vi "LET Output v3.vi"() -> ()   [LabVIEW 2010]
doc: "Cont(inuous) Acq(uire) & Chart (hw timed) demonstrates the hardware timed, non-buffered technique of data acquisition. The scan clock on the board controls acquisition timing. Acquired scans are read directly from the device's FIFO using AI Single Scan. \n\nThe acquisition is configured with no buffer, and the on-board scan clock started at the selected scan rate. In the first loop iteration, the newest (most recent) scan is read from the FIFO. In each subsequent loop iteration AI Single Scan is called to read the oldest scan from the FIFO. Then if a scan is missed because the acquisition does not keep up, an error message will be displayed, and the acquisition stopped. Each scan is plotted on the chart after it is read. \n\nA common reason to use non-buffered acquisition is that some kind of processing needs to be done for each data point. You will probably want to add more functions to the diagram to customize this VI for your application. The acquisition rate you can achieve depends on how much processing and display the VI must do. This VI calls a subVI named My Single-Scan Processing. Add whatever processing you need to this subVI, or replace it with one of your own. The data processing subVI also demonstrates how to use error clusters in your own subVIs, so they can be included in the error data flow chain.\n\nBefore running this VI, set the values of the controls on the front panel. Select Show Help Window from the Help menu to see a description of each control. If the values you select for all the controls are values you will usually use, select Make Current Values Default from the Operate menu and save the VI. Or, you may save individual control's default values by popping up on the control, selecting Data Operations, then selecting Make Current Value Default, and saving the VI."
uses:
  <instrlib>/agilent_b2900_series/Agilent B2900 Series/Public/Configure/Measurement/Configure Measurement (Current).vi
  <instrlib>/agilent_b2900_series/Agilent B2900 Series/Public/Configure/Measurement/Configure Measurement (Voltage).vi
  <vilib>/Analysis/Matrix/Numeric/Conversions/Matrix To Array - RM.vi
  <vilib>/Utility/file.llb/Write To Spreadsheet File (DBL).vi
  <instrlib>/agilent_b2900_series/Agilent B2900 Series/Agilent B2900 Series.lvlib
  <vilib>/Analysis/Matrix/NI_Matrix.lvlib
panel:
  out "Vds list":dbl[](array[numeric])
  out "Vgs list":dbl[](array[numeric])
  out "Real 2D Array":dbl[][](array[numeric])
  out "data matrix":dbl[][](array[numeric])
  out "Igs array 2":dbl[][](array[numeric])
  out "Vgs array 2":dbl[][](array[numeric])
  out "Vds array 2":dbl[][](array[numeric])
  out "Corrected PD current array 2":dbl[][](array[numeric])
  out "Ids array 2":dbl[][](array[numeric])
  out "corrected PD current array":dbl[](array[numeric])
  out "Vds array":dbl[](array[numeric])
  out "Ids array":dbl[](array[numeric])
  out "Vgs array":dbl[](array[numeric])
  out "Igs array":dbl[](array[numeric])
  in  "Tab Control":T1(tab)
  in  "keithley address":string="GPIB0::20::INSTR"
  in  "agilent address":refnum<visa-resource-name>="GPIB0::23::INSTR"
  in  "Initial Vds (V)\n(100 scans/sec)":sgl caption="Initial Vds (V)" format="%.2f"
  in  "Vds step (V)":sgl=1.0 format="%.2f"
  in  "Vds delay time":sgl=10.0 caption="Vds delay time (ms)" format="%.2f"
  in  "Vds delay after first value (ms)":sgl=10.0 format="%.2f"
  in  "Final Vds(V)":sgl=60.0 format="%.2f"
  in  "light emission ON/OFF":bool=TRUE
  in  "Vgs step (V)":sgl=20.0 format="%.2f"
  in  "Final Vgs (V)":sgl=60.0 format="%.2f"
  in  "Initial Vgs (V)":sgl format="%.2f"
  in  "Vgs hold time (ms)":i32=10
  in  "Compliance Voltage (channel 2)":dbl=60.0
  in  "Compliance Current (channel 1)":dbl=0.001
  in  "Compliance Voltage (channel 1)":dbl=60.0
  in  "Compliance Current (channel 2)":dbl=0.0001
  in  "keithley compliance limit":dbl(ring)=0.025 items=["25uA"=2.5e-05, "250uA"=0.00025, "2.5mA"=0.0025, "25mA"=0.025]
  in  "Loop":bool=TRUE
  in  "keithley current resolution":dbl=0.0001 format="%^.2e"
  in  "Current Auto Range Mode (0: Normal)":i32(ring) items=["Normal", "Resolution", "Speed"]
  in  "Voltage Auto Range Mode (0: Normal)":i32(ring) items=["Normal", "Resolution", "Speed"]
  in  "aperture time":dbl(ring)=-2.0 format="%.2f" items=["KE6485_VAL_RATE_FAST"=-1.0, "KE6485_VAL_RATE_MEDIUM"=-2.0, "KE6485_VAL_RATE_SLOW"=-3.0]
  in  "Auto Current NPLC (F: Disable)":bool
  in  "Current NPLC (0.1)":dbl=0.1
  in  "Auto Voltage NPLC(F: Disable)":bool
  in  "Voltage NPLC (0.1 PLC)":dbl=0.1
  out "Current Scan":cluster{dbl[], dbl[]}(graph)
  out "Applied Vds":sgl caption="current VDS (V)" format="%.2f"
  out "Applied Vgs":sgl caption="current VDS (V)" format="%.2f"
  out "Measured Ids":dbl format="%.2e"
  out "Measured Vds":dbl
  out "corrected PD current":dbl format="%^.2e"
  out "dark PD current (A)":dbl format="%^.2e"
  out "PD current":dbl format="%^.2e"
  out "Measured Igs":dbl
  out "Measured Vgs":dbl
  out "channel 2 status":bool
  out "channel 1 status":bool
  out "Current Scan 2":cluster{dbl[], dbl[]}(graph) caption="Current Scan"
  out "half  points":sgl
  out "Vds points":sgl
  out "Vgs points":sgl
  out "?":cluster{dbl[], dbl[]}[](graph)
  out "?":cluster{dbl[], dbl[]}[](graph)
  in  "error in keithley":errorcluster
  out "keithley address out":refnum<k15>
  out "error out keithley":errorcluster
  out "error out agilent":errorcluster
  out "Agilent address out":refnum<visa-resource-name>
  # "FET output v3"
  # "Drain-Source Setting"
  # "Gate Setting"
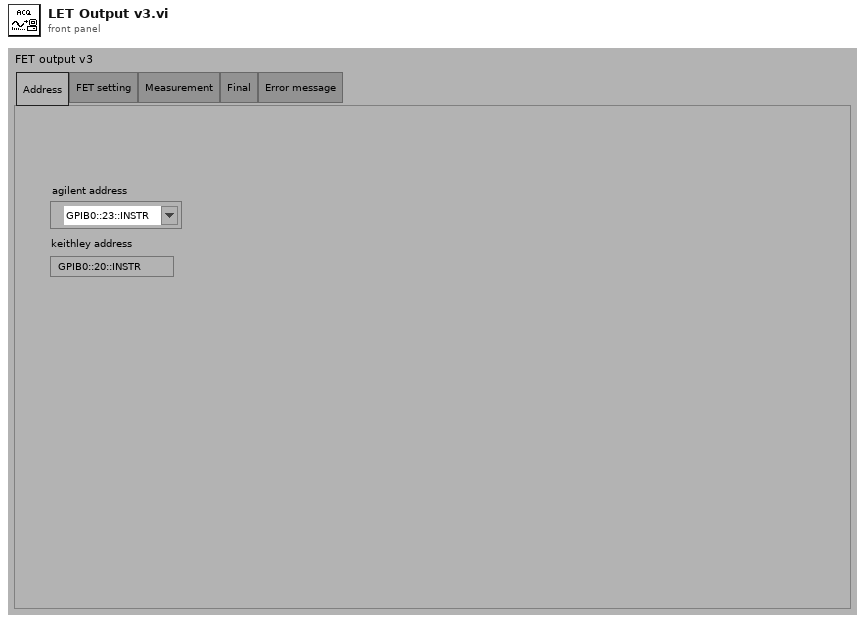
[diagram p1: front panel]
types:
  T1 = enum32{"Address", "FET setting", "Measurement", "Final", "Error message"}
  T2 = typedef "NI_Matrix.lvlib/RealMatrix.ctl" = dbl[][]
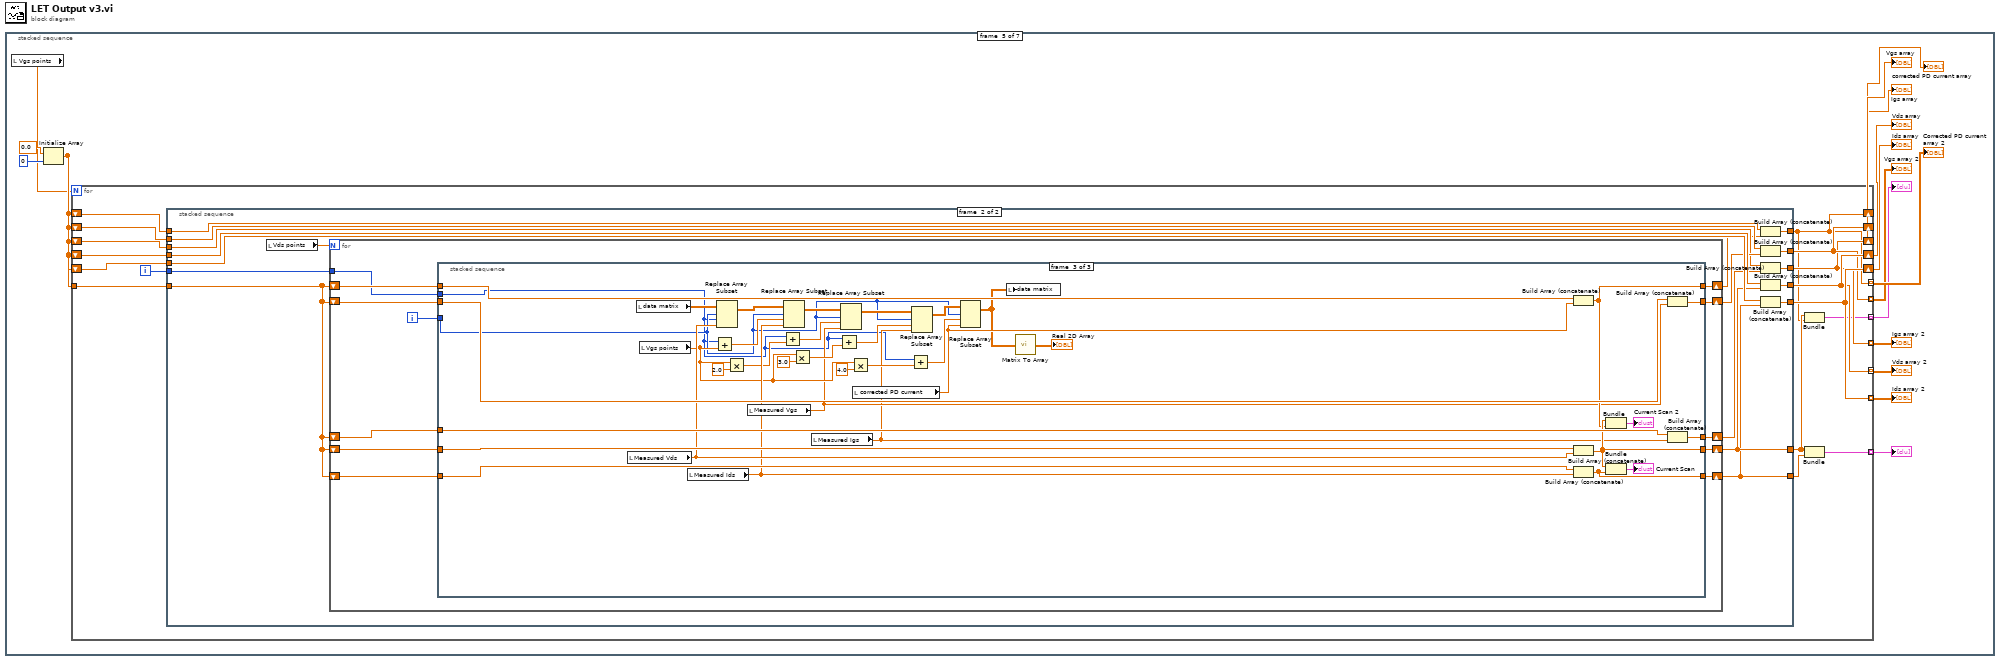
[diagram p0: block diagram]
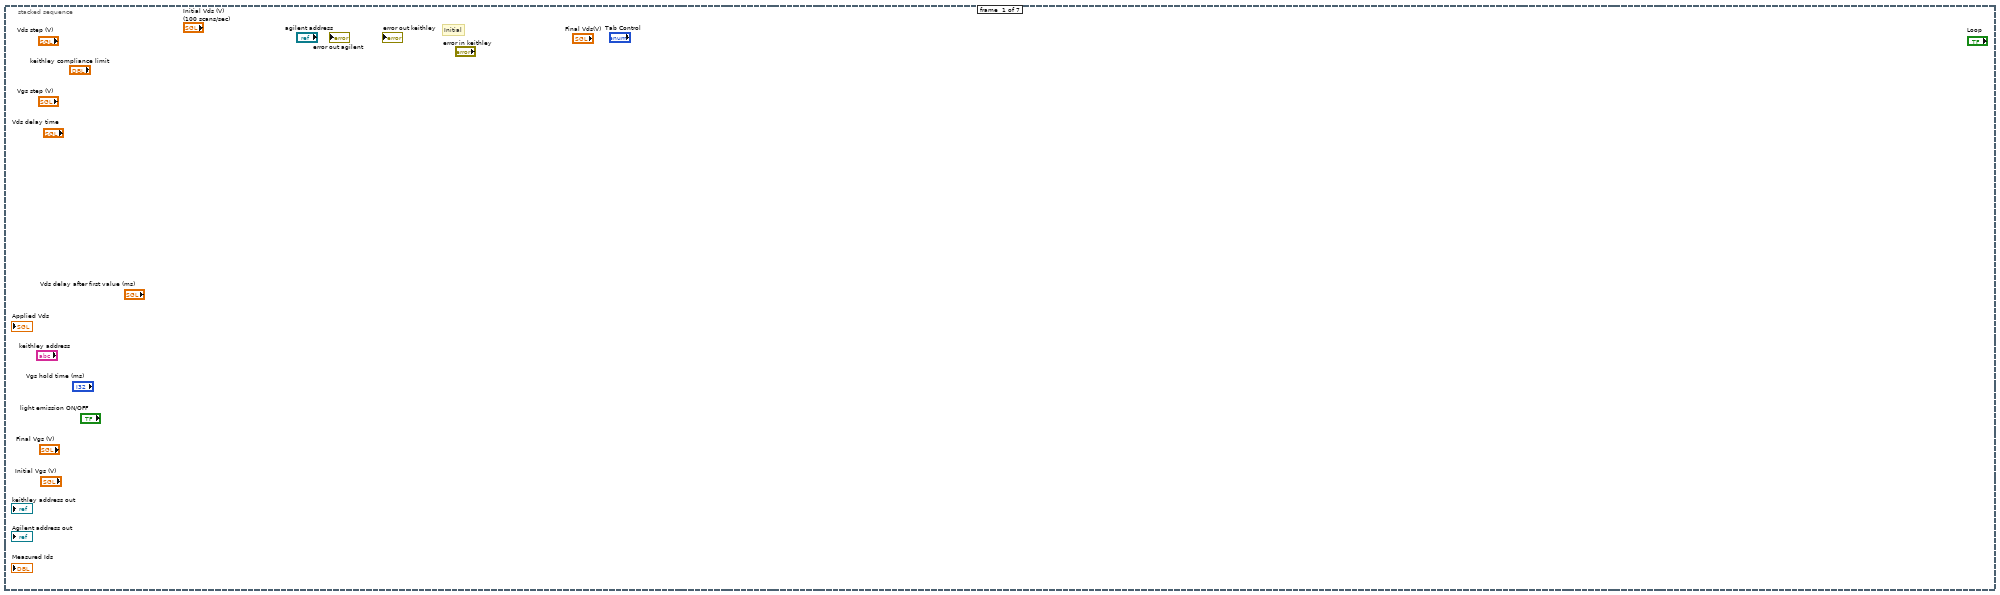
[diagram p2: hidden frame]
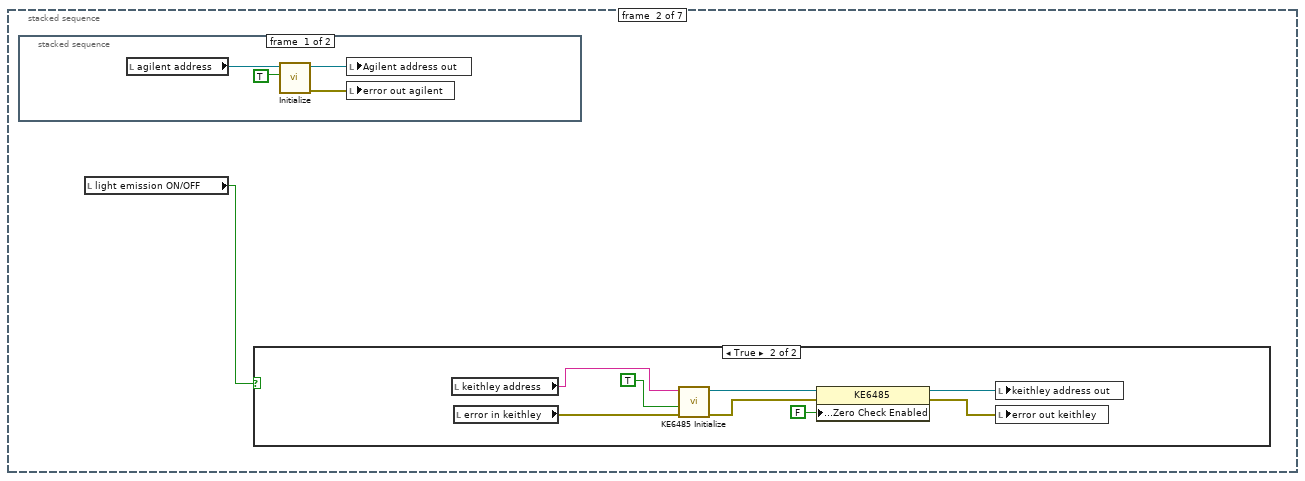
[diagram p3: hidden frame]
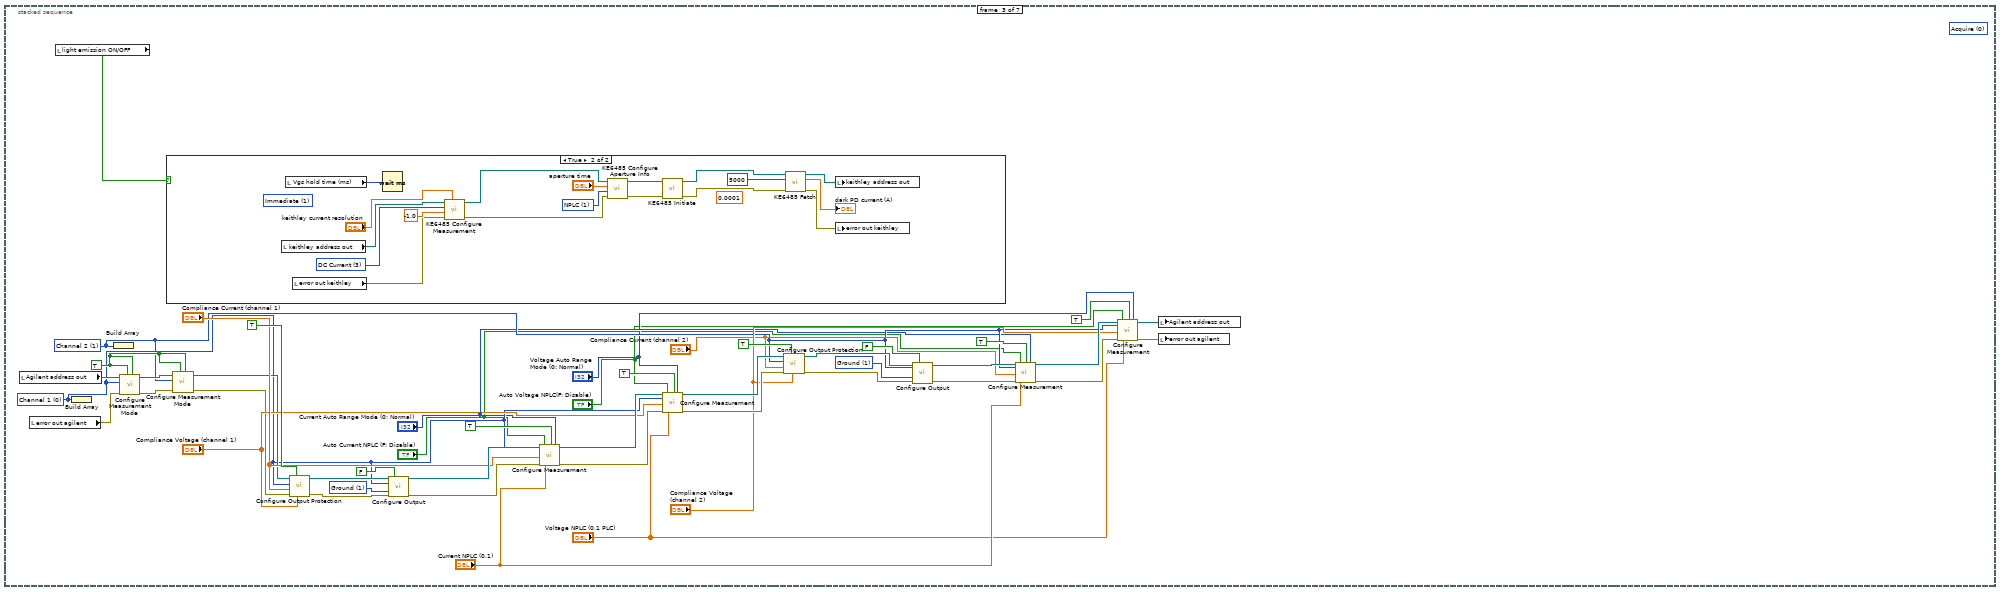
[diagram p6: hidden frame]
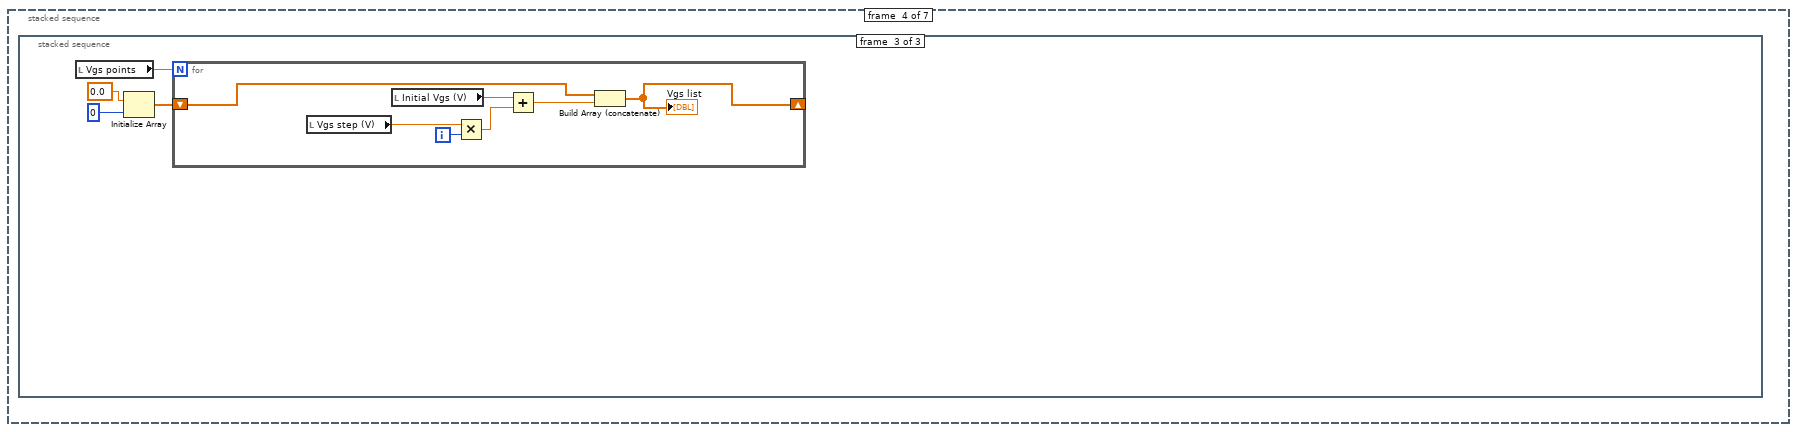
[diagram p8: hidden frame]
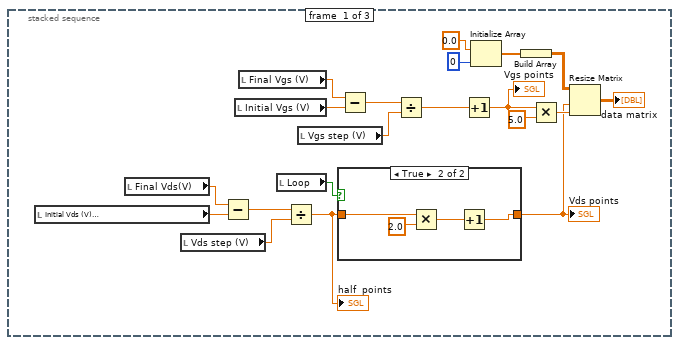
[diagram p9: hidden frame]
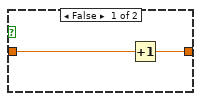
[diagram p10: hidden frame]
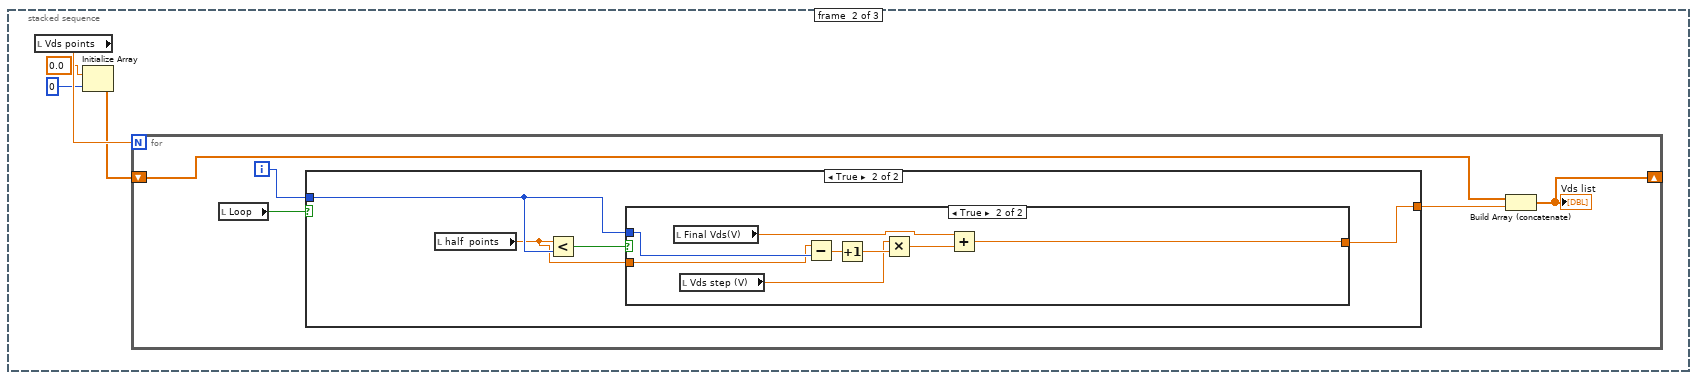
[diagram p11: hidden frame]
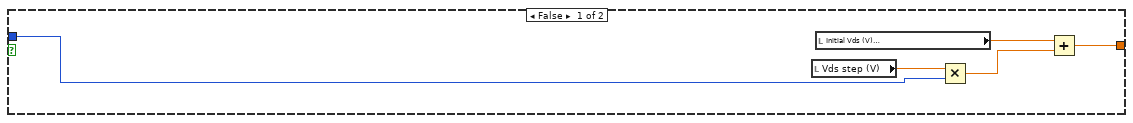
[diagram p12: hidden frame]
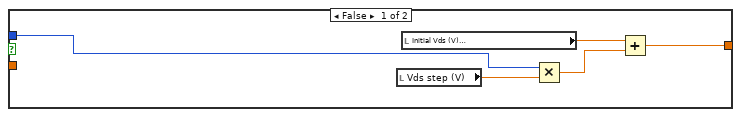
[diagram p13: hidden frame]
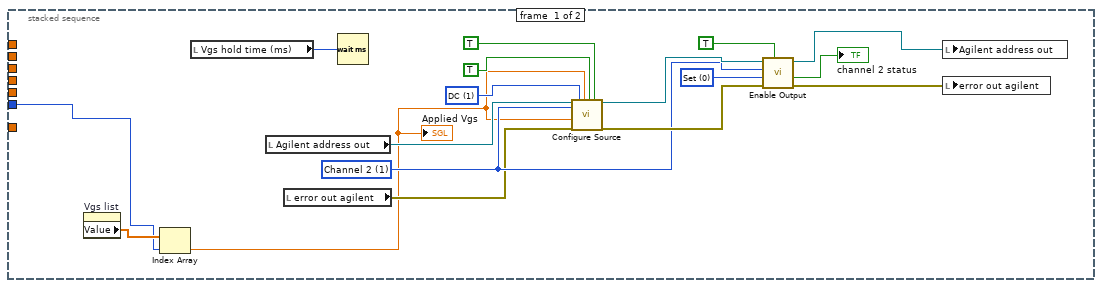
[diagram p14: hidden frame]
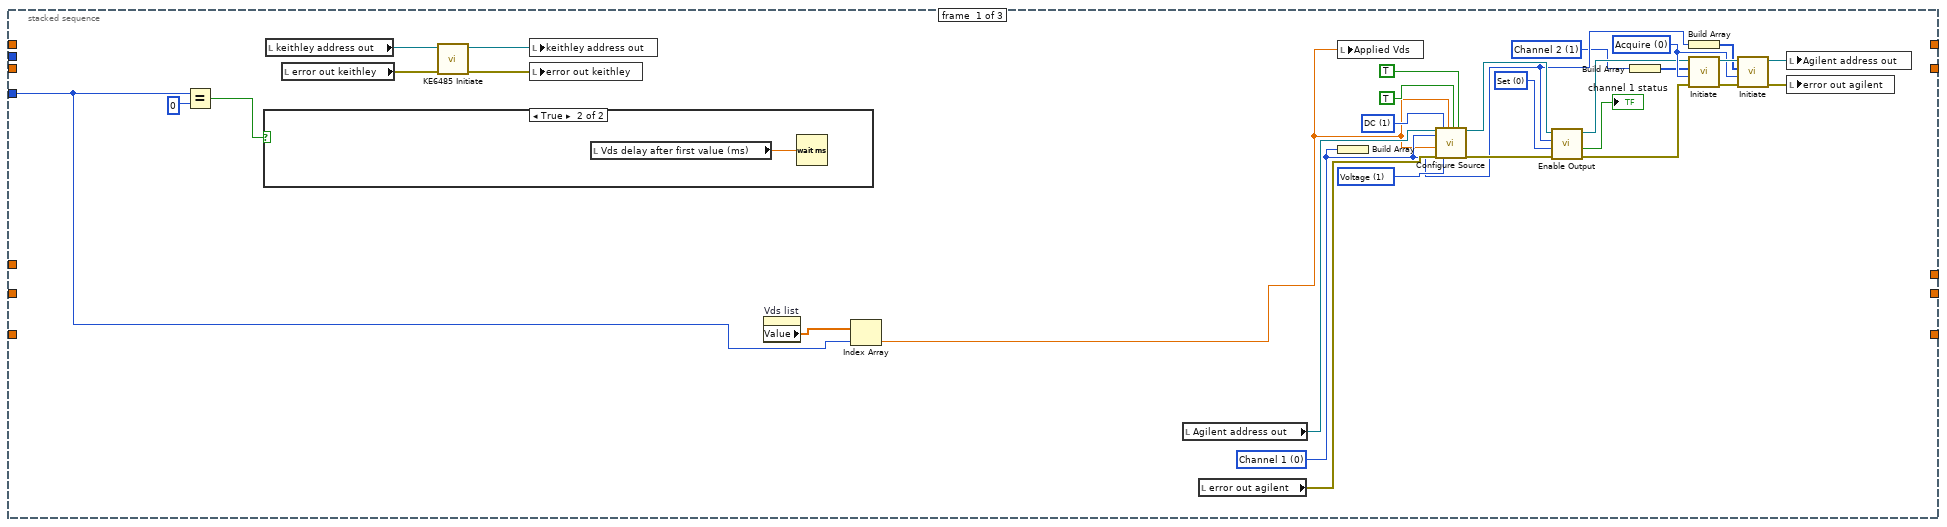
[diagram p15: hidden frame]
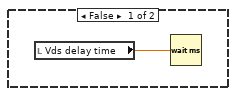
[diagram p16: hidden frame]
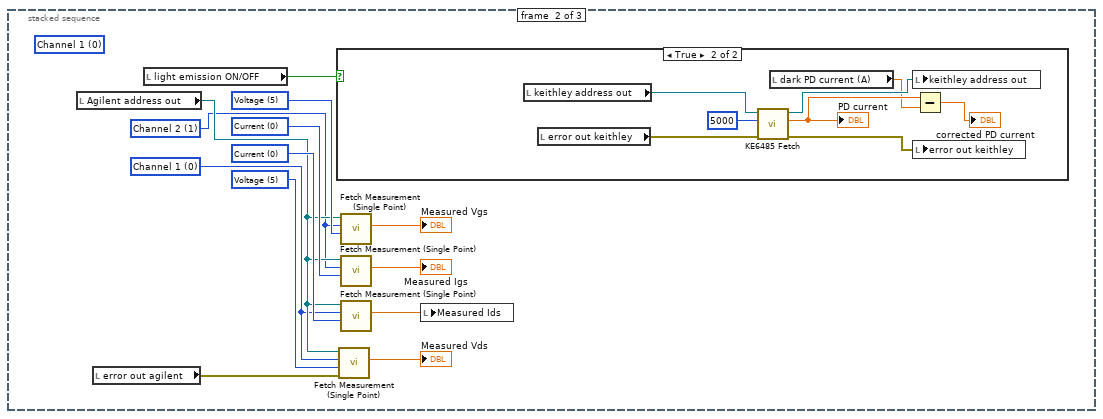
[diagram p17: hidden frame]
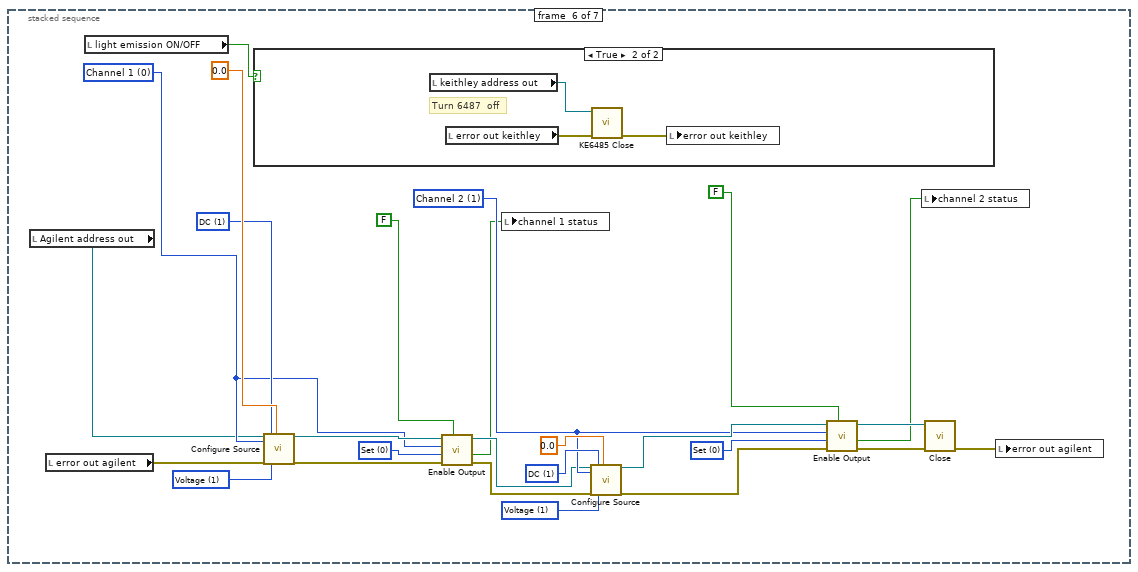
[diagram p19: hidden frame]
diagram:
  n1 = stacked-sequence {
    frame #0 {
      # "Initial"
    }
    frame #1 {
      n2 = stacked-sequence {
        frame #0 {
          n3 = local read "agilent address"() -> (w2:refnum<visa-resource-name>)
          n4 = call <instrlib>:"Initialize.vi"("ID Query (True)"=TRUE, "VISA resource name"=w2) -> ("error out"=w3:errorcluster, "VISA resource name out"=w4:refnum<visa-resource-name>)  [unwired: 8 in]
          n5 = local write "Agilent address out"(w4) -> ()
          n6 = local write "error out agilent"(w3) -> ()
        }
        frame #1 {
        }
      }
      n7 = local read "light emission ON/OFF"() -> (w1:bool)
      n8 = case shown="True" w1 {
        frame False {
        }
        frame True {
          n9 = local read "keithley address"() -> (w12:string)
          n10 = local read "error in keithley"() -> (w13:errorcluster)
          n11 = call <instrlib>:"KE6485 Initialize.vi"("error in (no error)"=w13, "reset device"=TRUE, "resource name"=w12) -> ("error out"=w10:errorcluster, "instrument handle out"=w9:refnum<k15>)  [unwired: 1 in, 6 out]
          n12 = property class="KE6485"(reference=w9, error in=w10, "System Settings:Zero Check Enabled"=FALSE) -> (reference out=w8:refnum<k15>, error out=w7:errorcluster)
          n13 = local write "keithley address out"(w8) -> ()
          n14 = local write "error out keithley"(w7) -> ()
        }
      }
    }
    frame #2 {
      (unwired) 0 items=["Acquire", "Transient", "Both"] ("Device Action (2: Both)")
      w30 = TRUE ("Enable Voltage Measurement (T: Enable)")
      w42 = 1 items=["Float", "Ground"] ("Low Terminal State (1: Ground)")
      w22 = 1 items=["Channel 1", "Channel 2"] ("Channel (0: Channel 1)")
      w52 = 1 items=["Float", "Ground"] ("Low Terminal State (1: Ground)")
      w23 = 0 items=["Channel 1", "Channel 2"] ("Channel (0: Channel 1)")
      n15 = local read "Agilent address out"() -> (w25:refnum<visa-resource-name>)
      n16 = local read "error out agilent"() -> (w27:errorcluster)
      n17 = local read "light emission ON/OFF"() -> (w59:bool)
      n18 = Build Array(w23) -> ()  [unwired: 1 out]
      n19 = Build Array(w22) -> ()  [unwired: 1 out]
      n20 = call <instrlib>:"Configure Measurement Mode.vi"("Enable Current Measurement (T: Enable)"=w30, "Enable Voltage Measurement (T: Enable)"=w30, "error in (no error)"=w27, "Channel (0: Channel 1)"=w23, "VISA resource name"=w25) -> ("error out"=w28:errorcluster, "VISA resource name out"=w29:refnum<visa-resource-name>)  [unwired: 5 in]
      n21 = case shown="True" w59 {
        frame False {
        }
        frame True {
          w65 = 1 items=["NPLC"=1] ("aperture time unit")
          (unwired) 0.0001 ("resolution (absolute)")
          (unwired) 1 items=["Immediate"=1, "Interval"=10, "Trigger Link 1"=1001, "Trigger Link 2"=1002, "Trigger Link 3"=1003, "Trigger Link 4"=1004, "Trigger Link 5"=1005, "Trigger Link 6"=1006] ("sample trigger")
          w75 = 3 items=["DC Volts"=1, "DC Current"=3, "2 Wire Resistance"=5, "Charge"=1004] ("measurement function")
          n22 = local read "keithley address out"() -> (w70:refnum<k15>)
          n23 = local read "Vgs hold time (ms)"() -> (w77:i32)
          n24 = local read "error out keithley"() -> (w69:errorcluster)
          n25 = Wait (ms)(milliseconds to wait=w77) -> ()  [unwired: 1 out]
          n26 = call <instrlib>:"KE6485 Configure Measurement.vi"("resolution (absolute)"="keithley current resolution", "error in (no error)"=w69, "range"=-1.0, "measurement function"=w75, "instrument handle"=w70) -> ("error out"=w64:errorcluster, "instrument handle out"=w63:refnum<k15>)  [unwired: 5 in]
          n27 = call <instrlib>:"KE6485 Configure Aperture Info.vi"("error in (no error)"=w64, "aperture time unit"=w65, "aperture time"="aperture time", "instrument handle"=w63) -> ("error out"=w61:errorcluster, "instrument handle out"=w62:refnum<k15>)  [unwired: 6 in]
          n28 = call <instrlib>:"KE6485 Initiate.vi"("error in (no error)"=w61, "instrument handle"=w62) -> ("error out"=w67:errorcluster, "instrument handle out"=w68:refnum<k15>)  [unwired: 8 in]
          n29 = call <instrlib>:"KE6485 Fetch.vi"("error in (no error)"=w67, "maximum time (ms)"=5000, "instrument handle"=w68) -> ("error out"=w72:errorcluster, "reading"=→"dark PD current (A)":dbl, "instrument handle out"=w71:refnum<k15>)  [unwired: 6 in]
          n30 = local write "keithley address out"(w71) -> ()
          n31 = local write "error out keithley"(w72) -> ()
        }
      }
      n32 = call <instrlib>:"Configure Measurement Mode.vi"("Enable Current Measurement (T: Enable)"=w30, "Enable Voltage Measurement (T: Enable)"=w30, "error in (no error)"=w28, "Channel (0: Channel 1)"=w22, "VISA resource name"=w29) -> ("error out"=w26:errorcluster, "VISA resource name out"=w24:refnum<visa-resource-name>)  [unwired: 5 in]
      n33 = call <instrlib>:"Configure Output Protection.vi"("Compliance Voltage (2 V)"="Compliance Voltage (channel 1)", "Enable Output Protection (T: Enable)"=TRUE, "error in (no error)"=w26, "Compliance Current (0.0001 A)"="Compliance Current (channel 1)", "Channel (0: Channel 1)"=w23, "VISA resource name"=w24) -> ("error out"=w54:errorcluster, "VISA resource name out"=w53:refnum<visa-resource-name>)  [unwired: 4 in]
      n34 = call <instrlib>:"Configure Output.vi"("VISA resource name"=w53, "Auto Output-Off (F: Disable)"=FALSE, "Channel (0: Channel 1)"=w23, "Low Terminal State (1: Ground)"=w52, "error in (no error)"=w54) -> ("VISA resource name out"=w50:refnum<visa-resource-name>, "error out"=w51:errorcluster)  [unwired: 9 in]
      n35 = call-poly <instrlib>:"Configure Measurement.vi"("VISA resource name"=w50, "Channel (0: Channel 1)"=w23, "Current Range (0.0001 A)"="Compliance Current (channel 1)", "error in (no error)"=w51, "Auto Current NPLC (F: Disable)"="Auto Current NPLC (F: Disable)", "Current NPLC (0.1)"="Current NPLC (0.1)", "Current Auto Range (T: Enable)"=TRUE, "Current Auto Range Mode (0: Normal)"="Current Auto Range Mode (0: Normal)") -> ("VISA resource name out"=w58:refnum<visa-resource-name>, "error out"=w57:errorcluster)  [unwired: 10 in]
      n36 = call-poly <instrlib>:"Configure Measurement.vi"("VISA resource name"=w58, "Channel (0: Channel 1)"=w23, "Voltage Range (2 V)"="Compliance Voltage (channel 1)", "error in (no error)"=w57, "Auto Voltage NPLC(F: Disable)"="Auto Voltage NPLC(F: Disable)", "Voltage NPLC (0.1 PLC)"="Voltage NPLC (0.1 PLC)", "Voltage Auto Range (T: Enable)"=TRUE, "Voltage Auto Range Mode (0: Normal)"="Voltage Auto Range Mode (0: Normal)") -> ("VISA resource name out"=w38:refnum<visa-resource-name>, "error out"=w37:errorcluster)  [unwired: 10 in]
      n37 = call <instrlib>:"Configure Output Protection.vi"("Compliance Voltage (2 V)"="Compliance Voltage (channel 2)", "Enable Output Protection (T: Enable)"=TRUE, "error in (no error)"=w37, "Compliance Current (0.0001 A)"="Compliance Current (channel 2)", "Channel (0: Channel 1)"=w22, "VISA resource name"=w38) -> ("error out"=w44:errorcluster, "VISA resource name out"=w43:refnum<visa-resource-name>)  [unwired: 4 in]
      n38 = call <instrlib>:"Configure Output.vi"("VISA resource name"=w43, "Auto Output-Off (F: Disable)"=FALSE, "Channel (0: Channel 1)"=w22, "Low Terminal State (1: Ground)"=w42, "error in (no error)"=w44) -> ("VISA resource name out"=w40:refnum<visa-resource-name>, "error out"=w41:errorcluster)  [unwired: 9 in]
      n39 = call-poly <instrlib>:"Configure Measurement.vi"("VISA resource name"=w40, "Channel (0: Channel 1)"=w22, "Current Range (0.0001 A)"="Compliance Current (channel 2)", "error in (no error)"=w41, "Auto Current NPLC (F: Disable)"="Auto Current NPLC (F: Disable)", "Current NPLC (0.1)"="Current NPLC (0.1)", "Current Auto Range (T: Enable)"=TRUE, "Current Auto Range Mode (0: Normal)"="Current Auto Range Mode (0: Normal)") -> ("VISA resource name out"=w48:refnum<visa-resource-name>, "error out"=w47:errorcluster)  [unwired: 10 in]
      n40 = call-poly <instrlib>:"Configure Measurement.vi"("VISA resource name"=w48, "Channel (0: Channel 1)"=w22, "Voltage Range (2 V)"="Compliance Voltage (channel 2)", "error in (no error)"=w47, "Auto Voltage NPLC(F: Disable)"="Auto Voltage NPLC(F: Disable)", "Voltage NPLC (0.1 PLC)"="Voltage NPLC (0.1 PLC)", "Voltage Auto Range (T: Enable)"=TRUE, "Voltage Auto Range Mode (0: Normal)"="Voltage Auto Range Mode (0: Normal)") -> ("VISA resource name out"=w21:refnum<visa-resource-name>, "error out"=w20:errorcluster)  [unwired: 10 in]
      n41 = local write "Agilent address out"(w21) -> ()
      n42 = local write "error out agilent"(w20) -> ()
    }
    frame #3 {
      n43 = stacked-sequence {
        frame #0 {
          n44 = local read "Initial Vds (V)\n(100 scans/sec)"() -> (w82:sgl)
          n45 = local read "Final Vds(V)"() -> (w81:sgl)
          n46 = local read "Vds step (V)"() -> (w83:sgl)
          n47 = Subtract(x=w81, y=w82) -> (x-y=w84:sgl)
          n48 = local read "Initial Vgs (V)"() -> (w95:sgl)
          n49 = local read "Final Vgs (V)"() -> (w94:sgl)
          n50 = local read "Loop"() -> (w80:bool)
          n51 = Divide(x=w84, y=w83) -> (x/y=w79:sgl)
          "half  points" <- w79
          n52 = local read "Vgs step (V)"() -> (w96:sgl)
          n53 = case shown="True" w80 {
            tunnel: w79 -> [w99 w103]
            tunnel: [w98 w101] -> w78
            frame False {
              n54 = Increment(x=w99) -> (x+1=w98:sgl)
            }
            frame True {
              n55 = Multiply(x=w103, y=sgl 2.0) -> (x*y=w100:sgl)
              n56 = Increment(x=w100) -> (x+1=w101:sgl)
            }
          }
          "Vds points" <- w78
          n57 = Subtract(x=w94, y=w95) -> (x-y=w92:sgl)
          n58 = Divide(x=w92, y=w96) -> (x/y=w93:sgl)
          n59 = Increment(x=w93) -> (x+1=w97:sgl)
          "Vgs points" <- w97
          n60 = Initialize Array(0.0 ("element"), 0 ("dimension size")) -> (w87:dbl[])
          n61 = Build Array(w87) -> (w88:T2)
          n62 = Multiply(x=w97, y=sgl 5.0) -> (x*y=w91:sgl)
          n63 = Resize Matrix(1:w91, 2:w78, 4:w88) -> (0:→"data matrix":T2)
        }
        frame #1 {
          n64 = local read "Vds points"() -> (w107:sgl)
          n65 = Initialize Array(0.0, 0) -> (w104:dbl[])
          n66 = for {
            N: w107 -> [_]
            shift-right: [w109] -> _
            shift-left: w104 -> [w110]
            i -> [w111]
            n67 = local read "Loop"() -> (w112:bool)
            n68 = case shown="True" w112 {
              tunnel: w111 -> [w115 w120]
              tunnel: [w113 w121] -> w108
              frame False {
                n69 = local read "Vds step (V)"() -> (w116:sgl)
                n70 = local read "Initial Vds (V)\n(100 scans/sec)"() -> (w114:sgl)
                n71 = Multiply(x=w116, y=w115) -> (x*y=w117:sgl)
                n72 = Add(x=w114, y=w117) -> (x+y=w113:sgl)
              }
              frame True {
                n73 = local read "half  points"() -> (w118:sgl)
                n74 = Less?(x=w118, y=w120) -> (x < y?=w119:bool)
                n75 = case shown="True" w119 {
                  tunnel: w120 -> [w124 w130]
                  tunnel: [w122 w127] -> w121
                  tunnel: w118 -> [_ w129]
                  frame False {
                    n76 = local read "Vds step (V)"() -> (w123:sgl)
                    n77 = local read "Initial Vds (V)\n(100 scans/sec)"() -> (w125:sgl)
                    n78 = Multiply(x=w124, y=w123) -> (x*y=w126:sgl)
                    n79 = Add(x=w125, y=w126) -> (x+y=w122:sgl)
                  }
                  frame True {
                    n80 = local read "Final Vds(V)"() -> (w131:sgl)
                    n81 = local read "Vds step (V)"() -> (w128:sgl)
                    n82 = Subtract(x=w129, y=w130) -> (x-y=w133:sgl)
                    n83 = Increment(x=w133) -> (x+1=w132:sgl)
                    n84 = Multiply(x=w128, y=w132) -> (x*y=w134:sgl)
                    n85 = Add(x=w131, y=w134) -> (x+y=w127:sgl)
                  }
                }
              }
            }
            n86 = Build Array (concatenate)(w110, w108) -> (w109:dbl[])
            "Vds list" <- w109
          }
        }
        frame #2 {
          n87 = local read "Vgs points"() -> (w138:sgl)
          n88 = Initialize Array(0.0, 0) -> (w135:dbl[])
          n89 = for {
            N: w138 -> [_]
            shift-right: [w144] -> _
            shift-left: w135 -> [w145]
            i -> [w140]
            n90 = local read "Vgs step (V)"() -> (w143:sgl)
            n91 = local read "Initial Vgs (V)"() -> (w142:sgl)
            n92 = Multiply(x=w143, y=w140) -> (x*y=w141:sgl)
            n93 = Add(x=w142, y=w141) -> (x+y=w139:sgl)
            n94 = Build Array (concatenate)(w145, w139) -> (w144:dbl[])
            "Vgs list" <- w144
          }
        }
      }
    }
    frame #4 {
      n95 = local read "Vgs points"() -> (w146:sgl)
      n96 = Initialize Array(0.0, 0) -> (w153:dbl[])
      n97 = for {
        N: w146 -> [_]
        shift-right: [w168] -> w158
        shift-left: w153 -> [w176]
        shift-right: [w169] -> w159
        shift-left: w153 -> [w175]
        shift-right: [w166] -> w157
        shift-left: w153 -> [w174]
        tunnel: [w173] -> w156 mode=indexing
        shift-right: [w165] -> w155
        shift-left: w153 -> [w172]
        shift-right: [w163] -> w154
        shift-left: w153 -> [w171]
        tunnel: w153 -> [w170]
        tunnel: [w169] -> w152 mode=indexing
        tunnel: [w163] -> w151 mode=indexing
        tunnel: [w168] -> w150 mode=indexing
        tunnel: [w166] -> w149 mode=indexing
        tunnel: [w165] -> w148 mode=indexing
        tunnel: [w162] -> w147 mode=indexing
        i -> [w177]
        n98 = stacked-sequence {
          tunnel: w177 -> [w179 w195]
          tunnel: w176 -> [_ w212]
          tunnel: w175 -> [_ w211]
          tunnel: [_ w206] -> w168
          tunnel: [_ w210] -> w169
          tunnel: w174 -> [_ w208]
          tunnel: [_ w207] -> w166
          tunnel: [_ w205] -> w164
          tunnel: [_ w204] -> w167
          tunnel: w172 -> [_ w203]
          tunnel: [_ w202] -> w165
          tunnel: [_ w200] -> w163
          tunnel: w171 -> [_ w198]
          tunnel: w170 -> [_ w196]
          frame #0 {
            w187 = 0 items=["Set", "Get"] ("Operation (0: Set)")
            w188 = 1 items=["Channel 1", "Channel 2"] ("Channel (0: Channel 1)")
            w191 = 1 items=["Pulse", "DC"] ("Source Shape (1: DC)")
            n99 = property on="Vgs list" class="Arr (strict)"() -> ("Value"=w180:dbl[])  [unwired: 2 in, 2 out]
            n100 = Index Array(array=w180, index=w179) -> (element=w178:dbl)
            "Applied Vgs" <- w178
            n101 = local read "Vgs hold time (ms)"() -> (w194:i32)
            n102 = local read "Agilent address out"() -> (w184:refnum<visa-resource-name>)
            n103 = local read "error out agilent"() -> (w183:errorcluster)
            n104 = Wait (ms)(milliseconds to wait=w194) -> ()  [unwired: 1 out]
            n105 = call <instrlib>:"Configure Source.vi"("VISA resource name"=w184, "Channel (0: Channel 1)"=w188, "Source Range (2)"=w178, "error in (no error)"=w183, "Source Shape (1: DC)"=w191, "Output Level (0)"=w178, "Source Auto Range (T: Enable)"=TRUE, "Enable Continuous Output (T: Enable)"=TRUE) -> ("VISA resource name out"=w193:refnum<visa-resource-name>, "error out"=w192:errorcluster)  [unwired: 10 in]
            n106 = call <instrlib>:"Enable Output.vi"("Enable Output (T: Enable)"=TRUE, "error in (no error)"=w192, "Operation (0: Set)"=w187, "Channel (0: Channel 1)"=w188, "VISA resource name"=w193) -> ("error out"=w182:errorcluster, "Output Enabled?"=→"channel 2 status":bool, "VISA resource name out"=w181:refnum<visa-resource-name>)  [unwired: 4 in]
            n107 = local write "Agilent address out"(w181) -> ()
            n108 = local write "error out agilent"(w182) -> ()
          }
          frame #1 {
            n109 = local read "Vds points"() -> (w197:sgl)
            n110 = for {
              N: w197 -> [_]
              shift-right: [w215] -> w204
              shift-left: w196 -> [w214]
              shift-right: [w217] -> w205
              shift-left: w196 -> [w216]
              shift-right: [w221] -> w209
              shift-left: w196 -> [w220]
              shift-right: [w219] -> w201
              shift-left: w196 -> [w218]
              shift-right: [w222] -> w199
              shift-left: w196 -> [w223]
              tunnel: w195 -> [w213]
              i -> [w224]
              n111 = stacked-sequence {
                tunnel: w224 -> [w226 _ w279]
                tunnel: w223 -> [_ _ w314]
                tunnel: [_ _ w303] -> w222
                tunnel: [_ _ w313] -> w221
                tunnel: w220 -> [_ _ w312]
                tunnel: [_ _ w311] -> w219
                tunnel: w218 -> [_ _ w310]
                tunnel: [_ _ w304] -> w217
                tunnel: w216 -> [_ _ w308]
                tunnel: [_ _ w306] -> w215
                tunnel: w214 -> [_ _ w307]
                tunnel: w213 -> [_ _ w278]
                frame #0 {
                  w240 = 0 items=["Acquire", "Transient", "Both"] ("Device Action (2: Both)")
                  w232 = 1 items=["Channel 1", "Channel 2"] ("Channel (0: Channel 1)")
                  w243 = 1 items=["Current", "Voltage"] ("Source Mode (1: Voltage)")
                  w246 = 1 items=["Pulse", "DC"] ("Source Shape (1: DC)")
                  w233 = 0 items=["Channel 1", "Channel 2"] ("Channel (0: Channel 1)")
                  w250 = 0 items=["Set", "Get"] ("Operation (0: Set)")
                  n112 = Equal?(x=w226, y=0) -> (x = y?=w253:bool)
                  n113 = case shown="True" w253 {
                    frame False {
                      n114 = local read "Vds delay time"() -> (w255:sgl)
                      n115 = Wait (ms)(milliseconds to wait=w255) -> ()  [unwired: 1 out]
                    }
                    frame True {
                      n116 = local read "Vds delay after first value (ms)"() -> (w256:sgl)
                      n117 = Wait (ms)(milliseconds to wait=w256) -> ()  [unwired: 1 out]
                    }
                  }
                  n118 = local read "keithley address out"() -> (w229:refnum<k15>)
                  n119 = local read "error out keithley"() -> (w228:errorcluster)
                  n120 = call <instrlib>:"KE6485 Initiate.vi"("error in (no error)"=w228, "instrument handle"=w229) -> ("error out"=w231:errorcluster, "instrument handle out"=w230:refnum<k15>)  [unwired: 8 in]
                  n121 = local write "keithley address out"(w230) -> ()
                  n122 = local write "error out keithley"(w231) -> ()
                  n123 = property on="Vds list" class="Arr (strict)"() -> ("Value"=w227:dbl[])  [unwired: 2 in, 2 out]
                  n124 = Index Array(array=w227, index=w226) -> (element=w225:dbl)
                  n125 = local read "Agilent address out"() -> (w248:refnum<visa-resource-name>)
                  n126 = local read "error out agilent"() -> (w247:errorcluster)
                  n127 = local write "Applied Vds"(w225) -> ()
                  n128 = Build Array(w233) -> ()  [unwired: 1 out]
                  n129 = call <instrlib>:"Configure Source.vi"("VISA resource name"=w248, "Channel (0: Channel 1)"=w233, "Source Range (2)"=w225, "error in (no error)"=w247, "Source Shape (1: DC)"=w246, "Source Mode (1: Voltage)"=w243, "Output Level (0)"=w225, "Source Auto Range (T: Enable)"=TRUE, "Enable Continuous Output (T: Enable)"=TRUE) -> ("VISA resource name out"=w252:refnum<visa-resource-name>, "error out"=w251:errorcluster)  [unwired: 9 in]
                  n130 = call <instrlib>:"Enable Output.vi"("error in (no error)"=w251, "Operation (0: Set)"=w250, "Channel (0: Channel 1)"=w233, "VISA resource name"=w252) -> ("error out"=w236:errorcluster, "Output Enabled?"=→"channel 1 status":bool, "VISA resource name out"=w237:refnum<visa-resource-name>)  [unwired: 5 in]
                  n131 = Build Array(w232) -> (w239:i32[])
                  n132 = Build Array(w233) -> (w238:i32[])
                  n133 = call <instrlib>:"Initiate.vi"("error in (no error)"=w236, "Device Action (2: Both)"=w240, "Channel List ({Channel1})"=w239, "VISA resource name"=w237) -> ("error out"=w242:errorcluster, "VISA resource name out"=w241:refnum<visa-resource-name>)  [unwired: 6 in]
                  n134 = call <instrlib>:"Initiate.vi"("error in (no error)"=w242, "Device Action (2: Both)"=w240, "Channel List ({Channel1})"=w238, "VISA resource name"=w241) -> ("error out"=w235:errorcluster, "VISA resource name out"=w234:refnum<visa-resource-name>)  [unwired: 6 in]
                  n135 = local write "Agilent address out"(w234) -> ()
                  n136 = local write "error out agilent"(w235) -> ()
                }
                frame #1 {
                  w258 = 1 items=["Channel 1", "Channel 2"] ("Channel (0: Channel 1)")
                  w259 = 0 items=["Channel 1", "Channel 2"] ("Channel (0: Channel 1)")
                  w264 = 0 items=["Current", "Resistance", "Source Output Setting", "Status", "Time", "Voltage"] ("Data Mode (5: Voltage)")
                  w265 = 5 items=["Current", "Resistance", "Source Output Setting", "Status", "Time", "Voltage"] ("Data Mode (5: Voltage)")
                  w267 = 0 items=["Current", "Resistance", "Source Output Setting", "Status", "Time", "Voltage"] ("Data Mode (5: Voltage)")
                  (unwired) 0 items=["Channel 1", "Channel 2"] ("Channel (0: Channel 1)")
                  w269 = 5 items=["Current", "Resistance", "Source Output Setting", "Status", "Time", "Voltage"] ("Data Mode (5: Voltage)")
                  n137 = local read "Agilent address out"() -> (w260:refnum<visa-resource-name>)
                  n138 = local read "error out agilent"() -> (w261:errorcluster)
                  n139 = local read "light emission ON/OFF"() -> (w257:bool)
                  n140 = case shown="True" w257 {
                    frame False {
                    }
                    frame True {
                      n141 = local read "keithley address out"() -> (w271:refnum<k15>)
                      n142 = local read "error out keithley"() -> (w270:errorcluster)
                      n143 = call <instrlib>:"KE6485 Fetch.vi"("error in (no error)"=w270, "maximum time (ms)"=5000, "instrument handle"=w271) -> ("error out"=w276:errorcluster, "reading"=w273:dbl, "instrument handle out"=w275:refnum<k15>)  [unwired: 6 in]
                      "PD current" <- w273
                      n144 = local read "dark PD current (A)"() -> (w272:dbl)
                      n145 = local write "keithley address out"(w275) -> ()
                      n146 = local write "error out keithley"(w276) -> ()
                      n147 = Subtract(x=w273, y=w272) -> (x-y=→"corrected PD current":dbl)
                    }
                  }
                  n148 = call <instrlib>:"Fetch Measurement (Single Point).vi"("error in (no error)"=w261, "Data Mode (5: Voltage)"=w269, "Channel (0: Channel 1)"=w259, "VISA resource name"=w260) -> ("Measurement"=→"Measured Vds":dbl)  [unwired: 5 in, 2 out]
                  n149 = call <instrlib>:"Fetch Measurement (Single Point).vi"("Data Mode (5: Voltage)"=w265, "Channel (0: Channel 1)"=w258, "VISA resource name"=w260) -> ("Measurement"=→"Measured Vgs":dbl)  [unwired: 6 in, 2 out]
                  n150 = call <instrlib>:"Fetch Measurement (Single Point).vi"("Data Mode (5: Voltage)"=w264, "Channel (0: Channel 1)"=w258, "VISA resource name"=w260) -> ("Measurement"=→"Measured Igs":dbl)  [unwired: 6 in, 2 out]
                  n151 = call <instrlib>:"Fetch Measurement (Single Point).vi"("Data Mode (5: Voltage)"=w267, "Channel (0: Channel 1)"=w259, "VISA resource name"=w260) -> ("Measurement"=w266:dbl)  [unwired: 6 in, 2 out]
                  n152 = local write "Measured Ids"(w266) -> ()
                }
                frame #2 {
                  n153 = local read "Measured Vds"() -> (w301:dbl)
                  n154 = local read "data matrix"() -> (w302:dbl[][])
                  n155 = local read "Vgs points"() -> (w285:sgl)
                  n156 = local read "Measured Ids"() -> (w298:dbl)
                  n157 = Add(x=w278, y=w285) -> (x+y=w299:sgl)
                  n158 = Replace Array Subset(array=w302, new element=w301, index (row)=w279, index (col)=w278) -> (w300:T2)
                  n159 = Multiply(x=w285, y=sgl 2.0) -> (x*y=w295:sgl)
                  n160 = local read "Measured Vgs"() -> (w284:dbl)
                  n161 = Add(x=w278, y=w295) -> (x+y=w296:sgl)
                  n162 = Replace Array Subset(array=w300, new element=w298, index (row)=w279, index (col)=w299) -> (w297:T2)
                  n163 = Multiply(x=w285, y=sgl 3.0) -> (x*y=w292:sgl)
                  n164 = local read "Measured Igs"() -> (w283:dbl)
                  n165 = Add(x=w278, y=w292) -> (x+y=w290:sgl)
                  n166 = Replace Array Subset(array=w297, new element=w284, index (row)=w279, index (col)=w296) -> (w293:T2)
                  n167 = Multiply(x=w285, y=sgl 4.0) -> (x*y=w288:sgl)
                  n168 = local read "corrected PD current"() -> (w282:dbl)
                  n169 = Add(x=w278, y=w288) -> (x+y=w286:sgl)
                  n170 = Replace Array Subset(array=w293, new element=w283, index (row)=w279, index (col)=w290) -> (w289:T2)
                  n171 = Replace Array Subset(array=w289, new element=w282, index (row)=w279, index (col)=w286) -> (w281:T2)
                  n172 = local write "data matrix"(w281) -> ()
                  n173 = call-poly <vilib>:"Matrix To Array.vi"("Real Matrix"=w281) -> ("Real 2D Array"=→"Real 2D Array":dbl[][])
                  n174 = Build Array (concatenate)(w314, w282) -> (w303:dbl[])
                  n175 = Build Array (concatenate)(w308, w301) -> (w304:dbl[])
                  n176 = Build Array (concatenate)(w307, w298) -> (w306:dbl[])
                  n177 = Bundle(w304, w303) -> (→"Current Scan 2":cluster{dbl[], dbl[]})  [unwired: 1 out]
                  n178 = Bundle(w304, w306) -> (→"Current Scan":cluster{dbl[], dbl[]})  [unwired: 1 out]
                  n179 = Build Array (concatenate)(w312, w284) -> (w313:dbl[])
                  n180 = Build Array (concatenate)(w310, w283) -> (w311:dbl[])
                }
              }
            }
            n181 = Build Array (concatenate)(w198, w199) -> (w200:dbl[])
            n182 = Build Array (concatenate)(w208, w209) -> (w207:dbl[])
            n183 = Build Array (concatenate)(w203, w201) -> (w202:dbl[])
            n184 = Build Array (concatenate)(w212, w205) -> (w206:dbl[])
            n185 = Build Array (concatenate)(w211, w204) -> (w210:dbl[])
          }
        }
        n186 = Bundle(w164, w163) -> (w162:cluster{dbl[], dbl[]})  [unwired: 1 out]
        n187 = Bundle(w164, w167) -> (w173:cluster{dbl[], dbl[]})  [unwired: 1 out]
      }
      "?" <- w156
      "Igs array" <- w155
      "Vgs array" <- w157
      "Ids array" <- w159
      "Vds array" <- w158
      "corrected PD current array" <- w154
      "Ids array 2" <- w152
      "Corrected PD current array 2" <- w151
      "Vds array 2" <- w150
      "Vgs array 2" <- w149
      "Igs array 2" <- w148
      "?" <- w147
    }
    frame #5 {
      w325 = 0 items=["Set", "Get"] ("Operation (0: Set)")
      w327 = 1 items=["Current", "Voltage"] ("Source Mode (1: Voltage)")
      w324 = 1 items=["Channel 1", "Channel 2"] ("Channel (0: Channel 1)")
      w328 = 1 items=["Pulse", "DC"] ("Source Shape (1: DC)")
      w333 = 0 items=["Set", "Get"] ("Operation (0: Set)")
      w335 = 1 items=["Current", "Voltage"] ("Source Mode (1: Voltage)")
      w332 = 0 items=["Channel 1", "Channel 2"] ("Channel (0: Channel 1)")
      w336 = 1 items=["Pulse", "DC"] ("Source Shape (1: DC)")
      n188 = local read "Agilent address out"() -> (w316:refnum<visa-resource-name>)
      n189 = local read "error out agilent"() -> (w315:errorcluster)
      n190 = local read "light emission ON/OFF"() -> (w340:bool)
      n191 = case shown="True" w340 {
        frame False {
        }
        frame True {
          # "Turn 6487  off"
          n192 = local read "keithley address out"() -> (w342:refnum<k15>)
          n193 = local read "error out keithley"() -> (w341:errorcluster)
          n194 = call <instrlib>:"KE6485 Close.vi"("error in (no error)"=w341, "instrument handle"=w342) -> ("error out"=w343:errorcluster)  [unwired: 9 out]
          n195 = local write "error out keithley"(w343) -> ()
        }
      }
      n196 = call <instrlib>:"Configure Source.vi"("VISA resource name"=w316, "Channel (0: Channel 1)"=w332, "error in (no error)"=w315, "Source Shape (1: DC)"=w336, "Source Mode (1: Voltage)"=w335, "Output Level (0)"=0.0) -> ("VISA resource name out"=w338:refnum<visa-resource-name>, "error out"=w334:errorcluster)  [unwired: 12 in]
      n197 = call <instrlib>:"Enable Output.vi"("Enable Output (T: Enable)"=FALSE, "error in (no error)"=w334, "Operation (0: Set)"=w333, "Channel (0: Channel 1)"=w332, "VISA resource name"=w338) -> ("error out"=w322:errorcluster, "Output Enabled?"=w318:bool, "VISA resource name out"=w323:refnum<visa-resource-name>)  [unwired: 4 in]
      n198 = local write "channel 1 status"(w318) -> ()
      n199 = call <instrlib>:"Configure Source.vi"("VISA resource name"=w323, "Channel (0: Channel 1)"=w324, "error in (no error)"=w322, "Source Shape (1: DC)"=w328, "Source Mode (1: Voltage)"=w327, "Output Level (0)"=0.0) -> ("VISA resource name out"=w330:refnum<visa-resource-name>, "error out"=w326:errorcluster)  [unwired: 12 in]
      n200 = call <instrlib>:"Enable Output.vi"("Enable Output (T: Enable)"=FALSE, "error in (no error)"=w326, "Operation (0: Set)"=w325, "Channel (0: Channel 1)"=w324, "VISA resource name"=w330) -> ("error out"=w321:errorcluster, "Output Enabled?"=w319:bool, "VISA resource name out"=w320:refnum<visa-resource-name>)  [unwired: 4 in]
      n201 = local write "channel 2 status"(w319) -> ()
      n202 = call <instrlib>:"Close.vi"("error in (no error)"=w321, "VISA resource name"=w320) -> ("error out"=w317:errorcluster)  [unwired: 9 in]
      n203 = local write "error out agilent"(w317) -> ()
    }
    frame #6 {
      n204 = local read "corrected PD current array"() -> (w345:dbl[])
      n205 = local read "Vgs array"() -> (w344:dbl[])
      n206 = local read "Vgs array"() -> (w347:dbl[])
      n207 = local read "Ids array"() -> (w348:dbl[])
      n208 = local read "Igs array"() -> (w346:dbl[])
      n209 = Two Button Dialog(message="Do you want to save the data?") -> (T button?=w349:bool)  [unwired: 2 out]
      n210 = case shown="True" w349 {
        tunnel: w347 -> [_ w356]
        tunnel: w348 -> [_ w355]
        tunnel: w346 -> [_ w353]
        tunnel: w345 -> [_ w352]
        tunnel: w344 -> [_ w354]
        frame False {
        }
        frame True {
          n211 = Build Array(w354, w355, w356, w353, w352) -> ()  [unwired: 1 out]
          n212 = local read "data matrix"() -> (w351:dbl[][])
          n213 = call-poly <vilib>:"Write To Spreadsheet File.vi"("transpose? (no:F)"=FALSE, "format (%.3f)"="%.4e", "append to file? (new file:F)"=FALSE, "2D data"=w351) -> ()  [unwired: 4 in, 1 out]
        }
      }
    }
  }
